vi "change channel select data typel test.vi"() -> ()   [LabVIEW 2013, in "current tag file io module tests.lvlib"]
uses:
  current tag file io module tests.lvlib
  module/configuration/tag configuration.ctl
  <vilib>/NI/Tag Bus Module Framework/channel/TBM channel.lvclass
  <vilib>/NI/Tag Bus/tag/Data Type.ctl
  module/configuration/current tag file io module configuration.lvclass/current tag file io module configuration.ctl
  <vilib>/NI/Tag Bus/tag/tag descriptor.lvclass/tag descriptor.ctl
  module/configuration/Read tags.vi
  <vilib>/NI/Tag Bus/tag/tag descriptor.lvclass
  module/configuration/current tag file io module configuration.lvclass
panel:
  out "Pass?":bool
  out "new data type":T1
  out "data type":T1
  out "data output 2":T1
  out "data output":T1
  out "new name":string
  out "output":string
  out "new tag":T2[](array[typedef])
  out "tag":T2[](array[typedef])
  out "error out":errorcluster
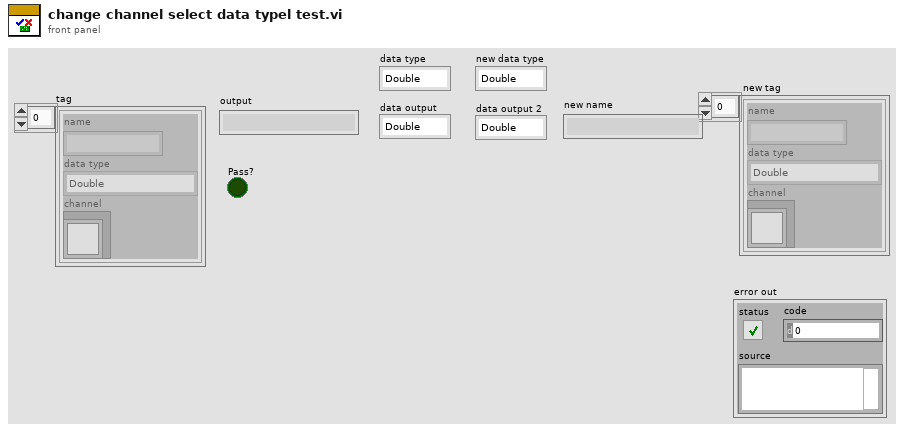
[diagram p1: front panel]
types:
  T1 = typedef "tag bus.lvlib/tag descriptor.lvclass/Data Type.ctl" = enum16{"Double", "Single", "I64", "I32", "I16", "I8", "U64", "U32", "U16", "U8", "Boolean", "String", "Array of Double", "Array of Single", "Array of I64", "Array of I32", "Array of I16", "Array of I8", "Array of U64", "Array of U32", "Array of U16", "Array of U8", "Array of Boolean", "Array of String"}
  T2 = typedef "current tag file io module configuration.lvclass/tag configuration.ctl" = cluster{"name":string, "data type":T1, "channel":refnum<class "TBM channel.lvclass">}
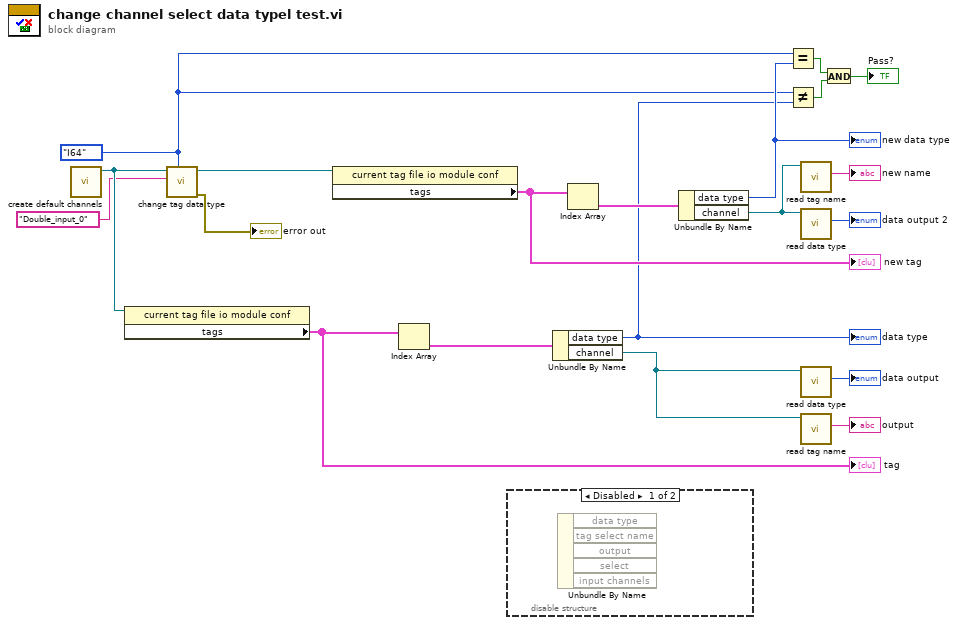
[diagram p0: block diagram]
diagram:
  w5 = Data_Type."I64" ("data type")
  n1 = call "create default channels.vi"() -> ("module"=w10:refnum<class "current tag file io module configuration.lvclass">)  [unwired: 7 in, 4 out]
  n2 = property class="current tag file io module conf"(reference=w10) -> ("tags"=w20:T2[])  [unwired: 1 in, 2 out]
  "tag" <- w20
  n3 = call "change tag data type.vi"("data type"=w5, "tag name"="Double_input_0" ("old name"), "current tag file io module configuration in"=w10) -> ("error out"=→"error out":errorcluster, "current tag file io module configuration out"=w9:refnum<class "current tag file io module configuration.lvclass">)  [unwired: 6 in, 1 out]
  n4 = property class="current tag file io module conf"(reference=w9) -> ("tags"=w15:T2[])  [unwired: 1 in, 2 out]
  "new tag" <- w15
  n5 = Index Array(array=w20) -> (element=w19:T2)  [unwired: 1 in]
  n6 = disable-structure shown="Disabled" {
    frame Disabled {
      n7 = Unbundle By Name() -> ()  [unwired: 1 in, 5 out]
    }
    frame Enabled {
    }
  }
  n8 = Unbundle By Name(w19) -> ("data type"=w4:T1, "channel"=w13:refnum<class "TBM channel.lvclass">)
  "data type" <- w4
  n9 = Index Array(array=w15) -> (element=w17:T2)  [unwired: 1 in]
  n10 = Unbundle By Name(w17) -> ("data type"=w6:T1, "channel"=w11:refnum<class "TBM channel.lvclass">)
  "new data type" <- w6
  n11 = Equal?(x=w5, y=w6) -> (x = y?=w3:bool)
  n12 = Not Equal?(x=w5, y=w4) -> (x != y?=w2:bool)
  n13 = call <vilib>:"read tag name.vi"("system tag in"=w11) -> ("name"=→"new name":string)  [unwired: 8 in, 2 out]
  n14 = call <vilib>:"read data type.vi"("system tag in"=w11) -> ("data type"=→"data output 2":T1)  [unwired: 8 in, 2 out]
  n15 = call <vilib>:"read data type.vi"("system tag in"=w13) -> ("data type"=→"data output":T1)  [unwired: 8 in, 2 out]
  n16 = call <vilib>:"read tag name.vi"("system tag in"=w13) -> ("name"=→"output":string)  [unwired: 8 in, 2 out]
  n17 = And(x=w3, y=w2) -> (x .and. y?=→"Pass?":bool)
